vi "2P power2angle convertor.vi"(8 "Error In":errorcluster, 10 "power(mW)":dbl format="%#_13g") -> (0 "Error Out":errorcluster, 2 "angle":dbl)   [LabVIEW 2018]
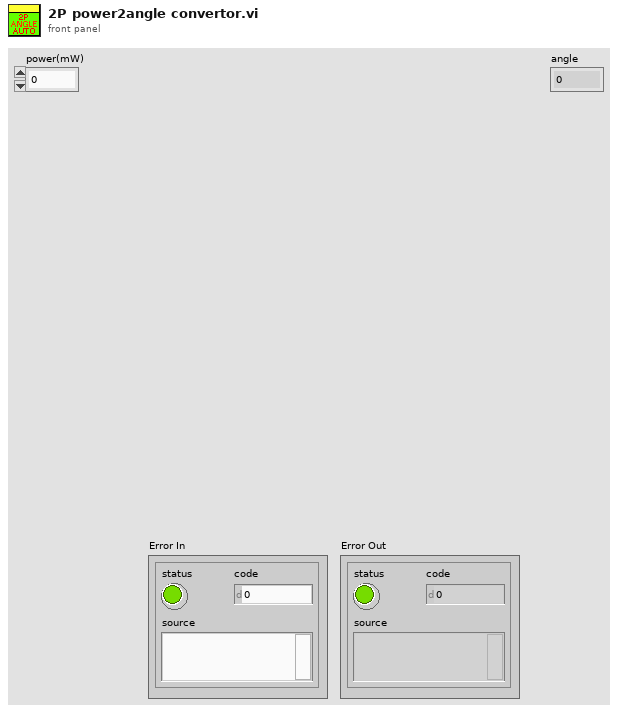
[diagram p1: front panel]
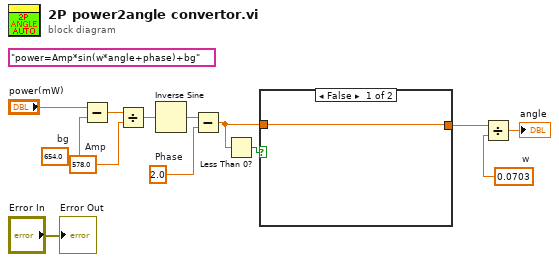
[diagram p0: block diagram]
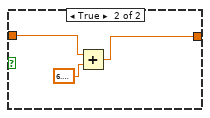
[diagram p2: hidden frame]
diagram:
  w5 = 654.0  # bg
  w9 = 0.0703  # w
  w10 = 2.0  # Phase
  w13 = 578.0  # Amp
  (unwired) "power=Amp*sin(w*angle+phase)+bg"
  n1 = Subtract(x="power(mW)", y=w5) -> (x-y=w4:dbl)
  n2 = Divide(x=w4, y=w13) -> (x/y=w12:dbl)
  n3 = Inverse Sine(1:w12) -> (0:w11:dbl)
  n4 = Subtract(x=w11, y=w10) -> (x-y=w2:dbl)
  n5 = Less Than 0?(x=w2) -> (x < 0?=w3:bool)
  n6 = case shown="False" w3 {
    tunnel: w2 -> [w14 w16]
    tunnel: [w14 w15] -> w1
    frame False {
    }
    frame True {
      n7 = Add(x=w16, y=6.283185307179586) -> (x+y=w15:dbl)
    }
  }
  n8 = Divide(x=w1, y=w9) -> (x/y=→"angle":dbl)
  "Error Out" <- "Error In"
